vi "UI.vi"() -> ()   [LabVIEW 2018]
uses:
  lib/Tango/SubVIs/AxisControl.ctl
  <vilib>/MakerHub/LINX/Public/Utilities/Open Serial.vi
  lib/Olympus IX BX Series/Olympus IX BX Series.lvlib
  <vilib>/MakerHub/LINX/LMH-LINX.lvlib
  lib/SOLA/LabVIEW 2015 Library (32bit)/LumencorDLL32/LumencorDLL32.lvlib
panel:
  in  "SOLA COM Port":u32=5 max=10 step=1
  in  "Light Source":u16(ring) items=["BF - Lamp", "SOLA"]
  out "error out":errorcluster
  in  "Flush\nReagent":u16
  in  "Flush":bool
  in  "Pump Cycles":dbl=20.0
  in  "Frequency":dbl=50.0 format="%#_3f"
  in  "Pump On":bool
  in  "Feed On":bool
  in  "Feed Cycles":dbl=20.0
  in  "Feed\nReagent":u16=2
  in  "Ring":u16
  in  "All Rings":bool
  in  "Direction (1: Down)":enum16{"Up", "Down", "Abs"}(ring)=enum."Abs"
  in  "Step (0.0 um)":dbl format="%.1f"
  in  "Filter":enum32{"", "BF", "UV", "GFP", "YFP", "RFP"}(ring)=enum."RFP"
  in  "Prism Position (1: Bi)":enum16{"Bi", "Side"}(ring)=enum."Side"
  in  "Shutter":bool
  in  "Objective":T1(ring)=enum."x 4"
  in  "Intensity [%]":dbl(slide) scale=0.0..100.0 scale format="%.1f"
  in  "Enable Lamp":bool
  in  "Lamp Type (0: Transmitted)":enum16{"Transmitted", "Reflected"}(ring)
  in  "stop":bool
  in  "Valve Port (Arduino)":refnum<visa-resource-name>="COM7"
  in  "IX 81 Port (IX2 UCB)":refnum<visa-resource-name>="IX2-UCB"
  out "Upper Limit":dbl
  out "Lower Limit":dbl
  in  "Move absolute":bool
  in  "Destination [mm]":dbl[](array[numeric]) format="%_6g"
  in  "Manual Control":T2[](array[typedef])
  in  "Step Width [mm]":dbl=1.0 min=0.0 format="%_6f"
  out "Position":dbl[](array[numeric]) format="%_6f"
  in  "TANGO COM Port":refnum<visa-resource-name>="COM4"
  # "Valve Functions"
  # "Initialization"
  # "Microscope"
  # "Stage"
  # "X"
  # "Y"
  # "Z"
  # "A"
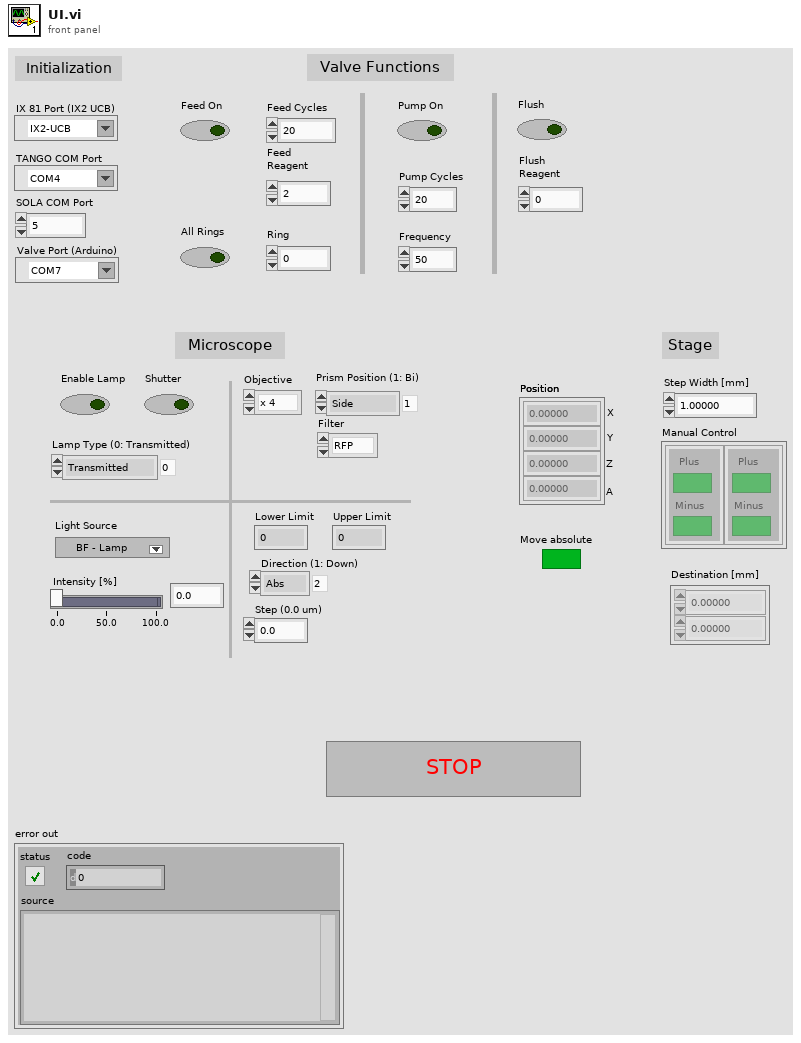
[diagram p1: front panel]
types:
  T1 = enum16{"", "x 4", "x 10", "x 20", "x 40", "x 100"}
  T2 = typedef "AxisControl.ctl" = cluster{"Plus":bool, "Minus":bool}
  T3 = typedef "LMH-LINX.lvlib/LINX Ref.ctl" = cluster{"IO":T4, "Interface":T5, "LINX Device Config":T6}
  T4 = typedef "LMH-LINX.lvlib/Platform.ctl" = enum16{"Remote", "Local"}
  T5 = typedef "LMH-LINX.lvlib/Interface.ctl" = enum16{"Serial", "TCP"}
  T6 = typedef "LMH-LINX.lvlib/Device.lvlib/LINX Device Config.ctl" = cluster{"Interface":T5, "COM Port":refnum<visa-resource-name>, "TCP Configuration":T7, "Device Family":u8, "Device ID":u8, "Device Name":string, "TCP Ref":refnum<k5>, "Channels":T8}
  T7 = typedef "LMH-LINX.lvlib/Device.lvlib/TCP Config.ctl" = cluster{"IP Address":string, "Port":u16}
  T8 = typedef "LMH-LINX.lvlib/Channels.ctl" = cluster{"DI":u8[], "DO":u8[], "AI":u8[], "AO":u8[], "PWM":u8[], "QE":u8[], "UART":u8[], "I2C 2":u8[], "SPI":u8[], "CAN":u8[], "Servo":u8[], "AI Ref (V)":dbl, "AI Resolution (Bits)":u8, "AO Ref (V)":dbl, "AO Resolution (Bits)":u8}
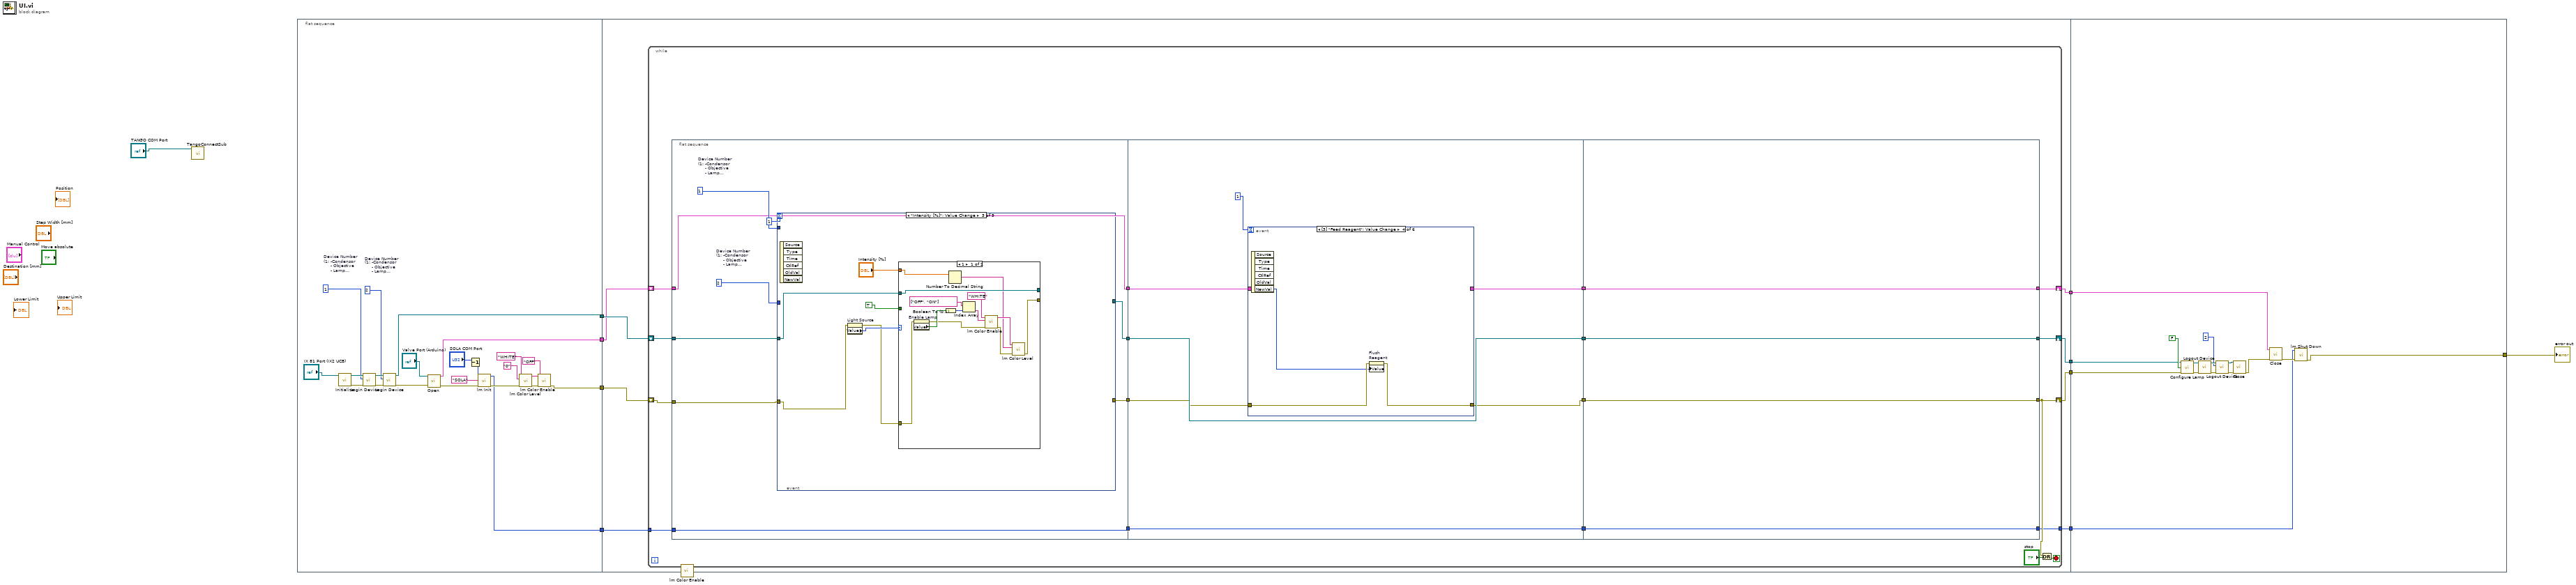
[diagram p0: block diagram]
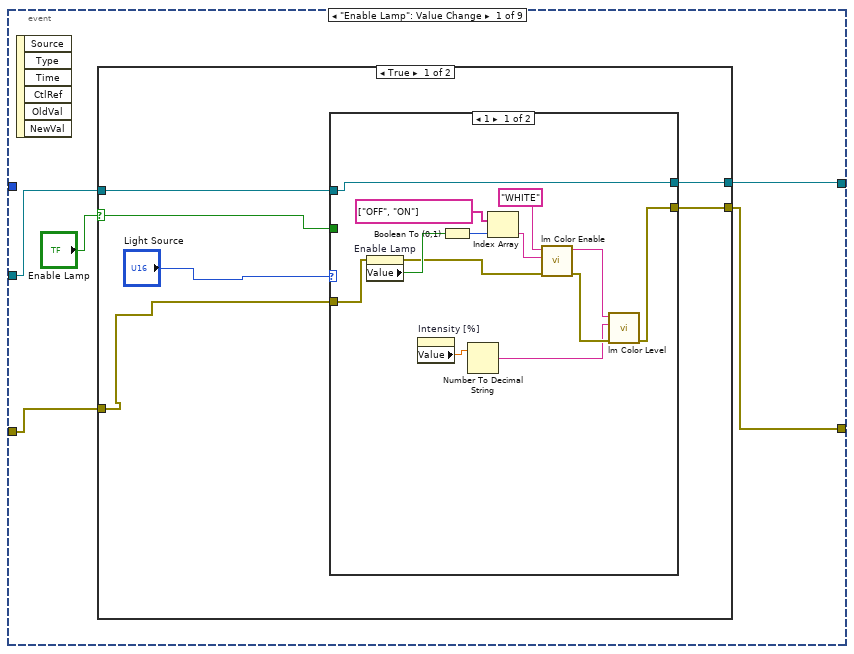
[diagram p2: hidden frame]
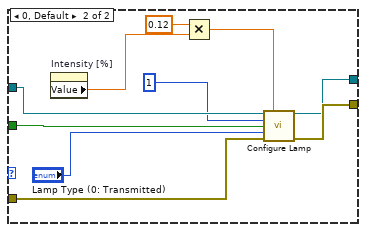
[diagram p3: hidden frame]
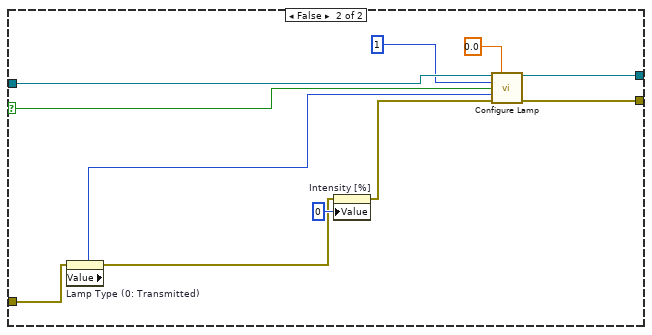
[diagram p4: hidden frame]
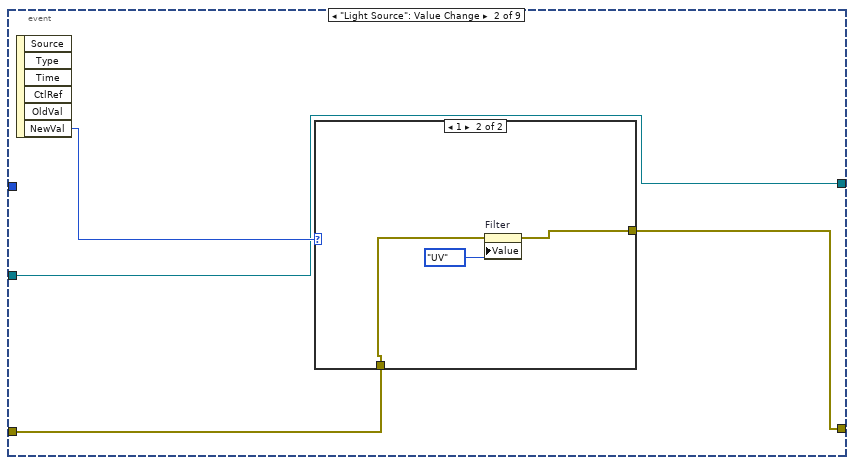
[diagram p5: hidden frame]
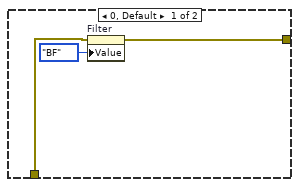
[diagram p6: hidden frame]
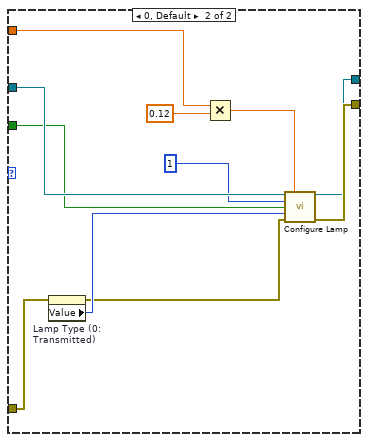
[diagram p7: hidden frame]
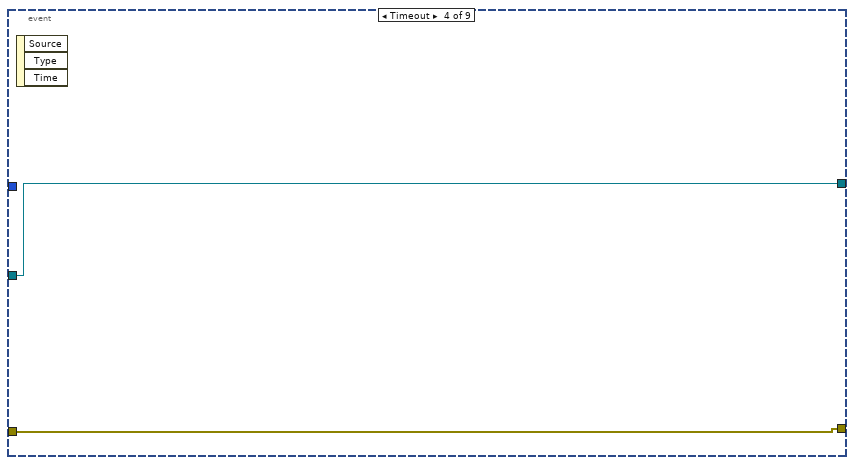
[diagram p8: hidden frame]
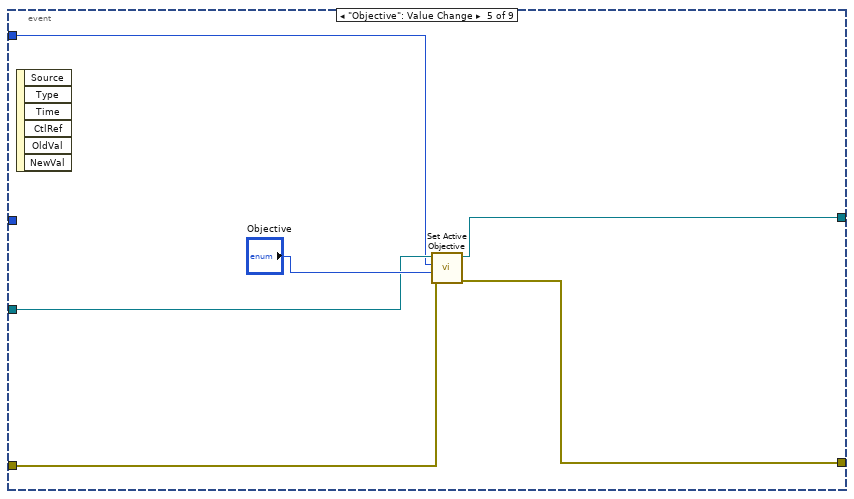
[diagram p9: hidden frame]
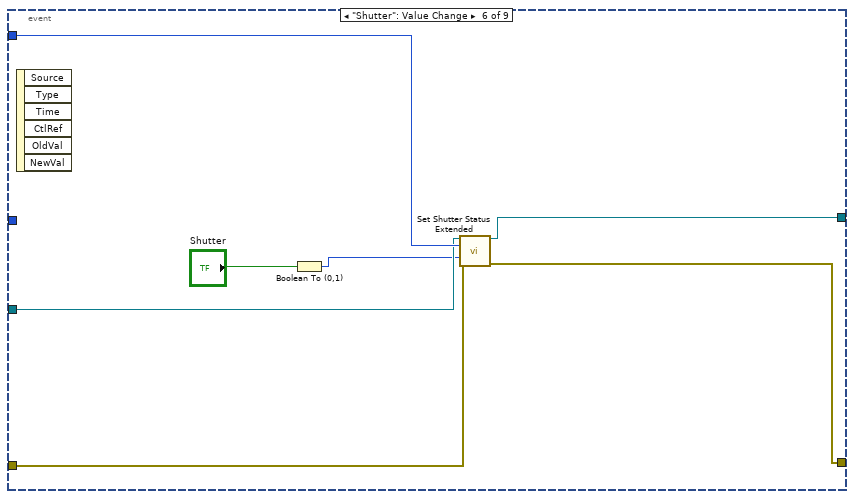
[diagram p10: hidden frame]
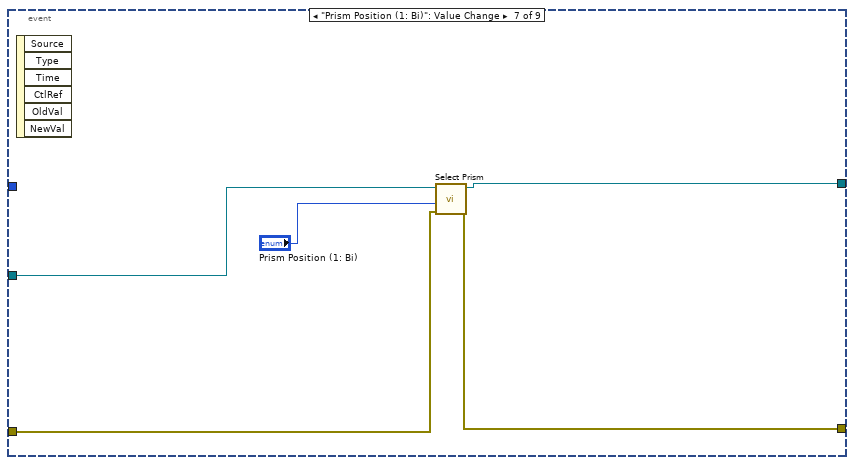
[diagram p11: hidden frame]
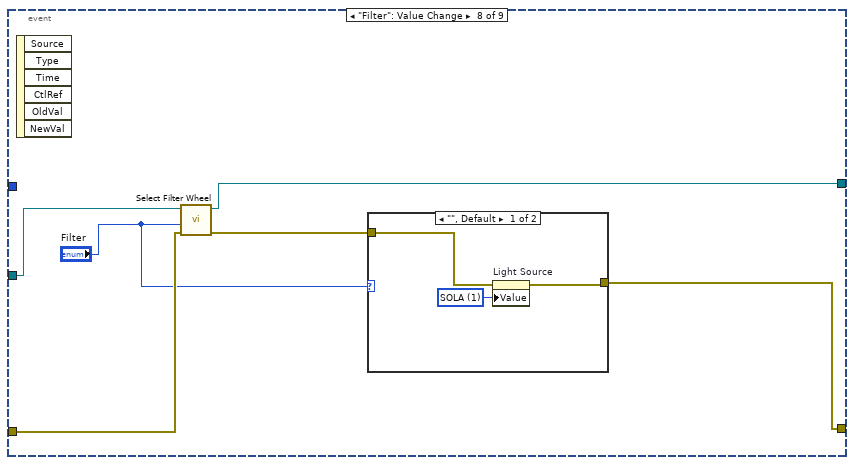
[diagram p12: hidden frame]
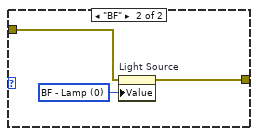
[diagram p13: hidden frame]
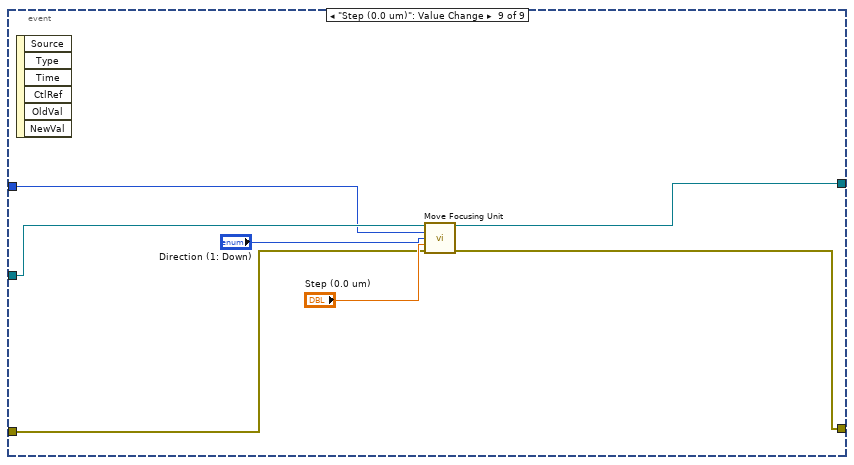
[diagram p14: hidden frame]
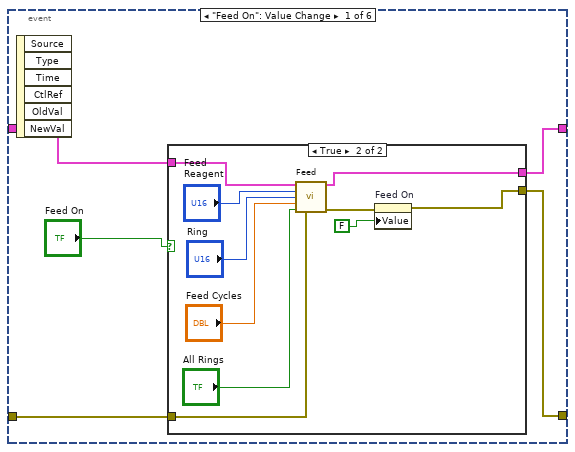
[diagram p15: hidden frame]
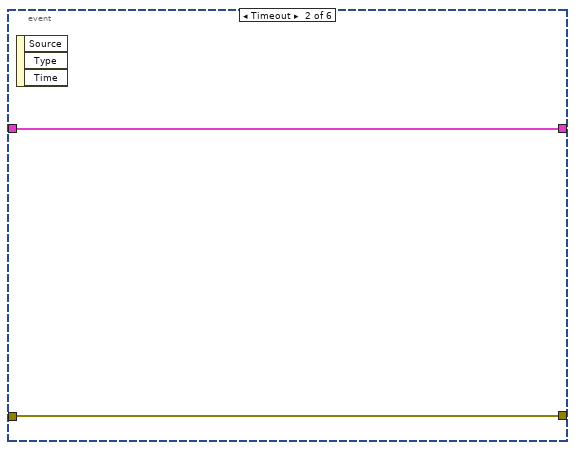
[diagram p17: hidden frame]
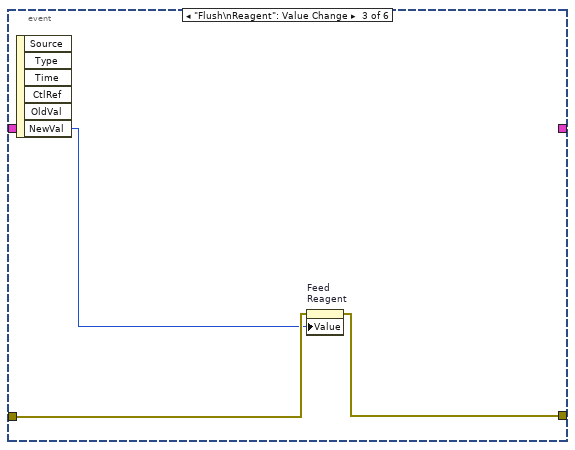
[diagram p18: hidden frame]
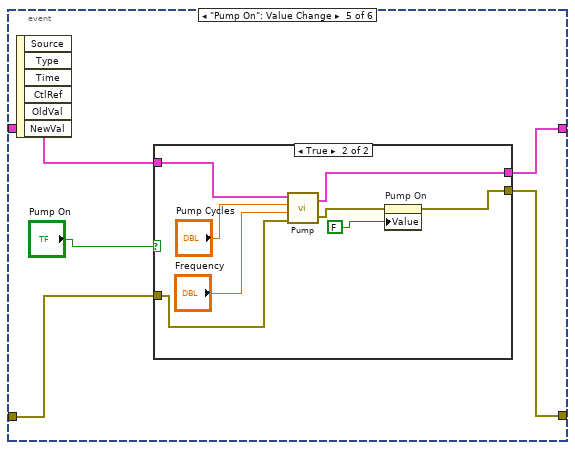
[diagram p19: hidden frame]
diagram:
  n1 = call "TangoConnectSub.vi"("VISA Refnum in"="TANGO COM Port") -> ()  [unwired: 8 in, 3 out]
  n2 = flat-sequence {
    tunnel: [w24] -> w9
    tunnel: [w23] -> w8
    tunnel: [w13] -> w7
    tunnel: [w12] -> w2
    tunnel: w9 -> [w41]
    tunnel: w8 -> [w39]
    tunnel: w7 -> [w40]
    tunnel: [w38] -> w6
    tunnel: [w37] -> w5
    tunnel: [w36] -> w4
    tunnel: w2 -> [w35]
    tunnel: [w34] -> w1
    tunnel: w6 -> [w261]
    tunnel: w5 -> [w260]
    tunnel: w4 -> [w259]
    tunnel: [w256] -> w3
    tunnel: w1 -> [w257]
    frame #0 {
      w26 = 2  # Device Number (1: -Condensor      - Objective      - Lamp      - Shutter 2: - Z-Motion    - Autofocus)
      w25 = 1  # Device Number (1: -Condensor      - Objective      - Lamp      - Shutter 2: - Z-Motion    - Autofocus)
      n3 = call "Initialize.vi"("VISA Resource Name"="IX 81 Port (IX2 UCB)") -> ("VISA Resource Name Out"=w32:refnum<visa-resource-name>, "error out"=w31:errorcluster)  [unwired: 13 in]
      n4 = call "Login Device.vi"("error in (no error)"=w31, "Device Number (1)"=w25, "VISA Resource Name"=w32) -> ("error out"=w29:errorcluster, "VISA Resource Name Out"=w30:refnum<visa-resource-name>)  [unwired: 7 in]
      n5 = call "Login Device.vi"("error in (no error)"=w29, "Device Number (1)"=w26, "VISA Resource Name"=w30) -> ("error out"=w27:errorcluster, "VISA Resource Name Out"=w24:refnum<visa-resource-name>)  [unwired: 7 in]
      n6 = call-poly <vilib>:"Open.vi"("Error In"=w27, "Serial Port"="Valve Port (Arduino)") -> ("Error Out"=w22:errorcluster, "LINX Resource"=w23:T3)  [unwired: 7 in, 1 out]
      n7 = Decrement(x="SOLA COM Port") -> (x-1=w11:u32)
      n8 = call "lm Init.vi"("error in (no error)"=w22, "LETypeStr"="SOLA", "ComPort"=w11) -> ("error out"=w19:errorcluster, "function return"=w12:u32)  [unwired: 6 in, 1 out]
      n9 = call "lm Color Level.vi"("error in (no error)"=w19, "str_Level"="0", "str_Color"="WHITE") -> ("error out"=w15:errorcluster, "str_Color out"=w16:string)  [unwired: 6 in, 1 out]
      n10 = call "lm Color Enable.vi"("error in (no error)"=w15, "str_State"="OFF", "str_Color"=w16) -> ("error out"=w13:errorcluster)  [unwired: 6 in, 2 out]
    }
    frame #1 {
      n11 = while {
        shift-right: [w46] -> w36
        shift-left: w40 -> [w56]
        shift-right: [w53] -> w38
        shift-left: w39 -> [w54]
        shift-right: [w55] -> w37
        shift-left: w41 -> [w57]
        tunnel: w35 -> [w45]
        tunnel: [w42] -> w34
        stop <- w58 stop-if-true
        n12 = flat-sequence {
          tunnel: w57 -> [w65]
          tunnel: w56 -> [w64]
          tunnel: [w63] -> w52
          tunnel: [w62] -> w51
          tunnel: w54 -> [w61]
          tunnel: [w61] -> w50
          tunnel: w45 -> [w60]
          tunnel: [w60] -> w44
          tunnel: w52 -> [w196]
          tunnel: [w196] -> w49
          tunnel: w51 -> [w195]
          tunnel: [w194] -> w48
          tunnel: w50 -> [w198]
          tunnel: [w197] -> w47
          tunnel: w44 -> [w193]
          tunnel: [w193] -> w43
          tunnel: [w254] -> w55
          tunnel: w49 -> [w254]
          tunnel: [w255] -> w46
          tunnel: w48 -> [w255]
          tunnel: [w253] -> w53
          tunnel: w47 -> [w253]
          tunnel: w43 -> [w252]
          tunnel: [w252] -> w42
          frame #0 {
            w66 = 2  # Device Number (1: -Condensor      - Objective      - Lamp      - Shutter 2: - Z-Motion    - Autofocus)
            w67 = 1  # Device Number (1: -Condensor      - Objective      - Lamp      - Shutter 2: - Z-Motion    - Autofocus)
            n13 = event shown="[2] \"Intensity [%]\": Value Change" {
              selector: _ -> [_ _ _ _ _ _ _ _ _]
              dyn-events: _ -> [_ _ _ _ _ _ _ _ _]
              timeout: 1 -> [_ _ _ _ _ _ _ _ _]
              tunnel: w65 -> [w72 w114 w128 w155 w158 w167 w170 w177 w189]
              tunnel: w67 -> [_ _ _ _ w156 w168 _ _ _]
              tunnel: w66 -> [_ _ _ _ _ _ _ _ w188]
              tunnel: [w71 w115 _ w154 w160 w162 w172 w174 w186] -> w62
              tunnel: [w70 w114 _ w155 w161 w163 w173 w179 w187] -> w63
              tunnel: w64 -> [w69 w116 w126 w154 w157 w166 w171 w178 w190]
              event "Enable Lamp": Value Change {
                n14 = event-data() -> ()  [unwired: 1 in, 6 out]
                n15 = case shown="True" "Enable Lamp" {
                  selector: "Enable Lamp" -> [w76 w109]
                  tunnel: w72 -> [w79 w113]
                  tunnel: w69 -> [w75 w104]
                  tunnel: [w78 w112] -> w71
                  tunnel: [w77 w111] -> w70
                  frame True {
                    n16 = case shown="1" "Light Source" {
                      tunnel: w79 -> [w92 w102]
                      tunnel: w75 -> [w86 w101]
                      tunnel: [w80 w100] -> w78
                      tunnel: [w92 w99] -> w77
                      tunnel: w76 -> [_ w97]
                      frame 1 {
                        n17 = property on="Enable Lamp" class="Bool (strict)"(error in=w86) -> (error out=w85:errorcluster, "Value"=w88:bool)  [unwired: 1 in, 1 out]
                        n18 = property on="Intensity [%]" class="Slide (strict)"() -> ("Value"=w82:dbl)  [unwired: 2 in, 2 out]
                        n19 = Boolean To (0,1)(Boolean=w88) -> (0, 1=w87:i16)
                        n20 = Number To Decimal String(number=w82) -> (decimal integer string=w81:string)  [unwired: 1 in]
                        n21 = Index Array(array=string[] ["OFF", "ON"], index=w87) -> (element=w90:string)
                        n22 = call "lm Color Enable.vi"("error in (no error)"=w85, "str_State"=w90, "str_Color"="WHITE") -> ("error out"=w84:errorcluster, "str_Color out"=w83:string)  [unwired: 6 in, 1 out]
                        n23 = call "lm Color Level.vi"("error in (no error)"=w84, "str_Level"=w81, "str_Color"=w83) -> ("error out"=w80:errorcluster)  [unwired: 6 in, 2 out]
                      }
                      frame 0, Default {
                        n24 = property on="Intensity [%]" class="Slide (strict)"() -> ("Value"=w94:dbl)  [unwired: 2 in, 2 out]
                        n25 = Multiply(x=0.12, y=w94) -> (x*y=w96:dbl)
                        n26 = call "Configure Lamp.vi"("VISA Resource Name"=w102, "Lamp Intensity (1.0 V)"=w96, "Device Number (1)"=1, "Lamp Enabled (True)"=w97, "Lamp Type (0: Transmitted)"="Lamp Type (0: Transmitted)", "error in (no error)"=w101) -> ("VISA Resource Name Out"=w99:refnum<visa-resource-name>, "error out"=w100:errorcluster)  [unwired: 8 in]
                      }
                    }
                  }
                  frame False {
                    n27 = property on="Lamp Type (0: Transmitted)" class="Enum (strict)"(error in=w104) -> (error out=w103:errorcluster, "Value"=w105:enum16{"Transmitted", "Reflected"})  [unwired: 1 in, 1 out]
                    n28 = property on="Intensity [%]" class="Slide (strict)"(error in=w103, "Value"=u16 0 ("Intensity [%]")) -> (error out=w108:errorcluster)  [unwired: 1 in, 1 out]
                    n29 = call "Configure Lamp.vi"("VISA Resource Name"=w113, "Lamp Intensity (1.0 V)"=0.0, "Device Number (1)"=1, "Lamp Enabled (True)"=w109, "Lamp Type (0: Transmitted)"=w105, "error in (no error)"=w108) -> ("VISA Resource Name Out"=w111:refnum<visa-resource-name>, "error out"=w112:errorcluster)  [unwired: 8 in]
                  }
                }
              }
              event "Light Source": Value Change {
                n30 = event-data() -> ("NewVal"=w117:u16)  [unwired: 1 in, 5 out]
                n31 = case shown="1" w117 {
                  tunnel: w116 -> [w119 w122]
                  tunnel: [w118 w121] -> w115
                  frame 0, Default {
                    n32 = property on="Filter" class="Enum (strict)"(error in=w119, "Value"=enum32{"", "BF", "UV", "GFP", "YFP", "RFP"}."BF" ("Filter")) -> (error out=w118:errorcluster)  [unwired: 1 in, 1 out]
                  }
                  frame 1 {
                    n33 = property on="Filter" class="Enum (strict)"(error in=w122, "Value"=enum32{"", "BF", "UV", "GFP", "YFP", "RFP"}."UV" ("Filter")) -> (error out=w121:errorcluster)  [unwired: 1 in, 1 out]
                  }
                }
              }
              event "Intensity [%]": Value Change {
                n34 = event-data() -> ()  [unwired: 1 in, 6 out]
                n35 = property on="Light Source" class="Ring (strict)"(error in=w126) -> (error out=w125:errorcluster, "Value"=w129:u16)  [unwired: 1 in, 1 out]
                n36 = case shown="1" w129 {
                  tunnel: w128 -> [w142 w153]
                  tunnel: [w132 w152] -> _
                  tunnel: [w142 w151] -> _
                  tunnel: TRUE -> [_ w149]
                  tunnel: w125 -> [w131 w146]
                  tunnel: "Intensity [%]" -> [w130 w144]
                  frame 1 {
                    n37 = property on="Enable Lamp" class="Bool (strict)"(error in=w131) -> (error out=w136:errorcluster, "Value"=w138:bool)  [unwired: 1 in, 1 out]
                    n38 = Boolean To (0,1)(Boolean=w138) -> (0, 1=w137:i16)
                    n39 = Number To Decimal String(number=w130) -> (decimal integer string=w133:string)  [unwired: 1 in]
                    n40 = Index Array(array=string[] ["OFF", "ON"], index=w137) -> (element=w140:string)
                    n41 = call "lm Color Enable.vi"("error in (no error)"=w136, "str_State"=w140, "str_Color"="WHITE") -> ("error out"=w135:errorcluster, "str_Color out"=w134:string)  [unwired: 6 in, 1 out]
                    n42 = call "lm Color Level.vi"("error in (no error)"=w135, "str_Level"=w133, "str_Color"=w134) -> ("error out"=w132:errorcluster)  [unwired: 6 in, 2 out]
                  }
                  frame 0, Default {
                    n43 = property on="Lamp Type (0: Transmitted)" class="Enum (strict)"(error in=w146) -> (error out=w145:errorcluster, "Value"=w147:enum16{"Transmitted", "Reflected"})  [unwired: 1 in, 1 out]
                    n44 = Multiply(x=w144, y=0.12 ("x")) -> (x*y=w148:dbl)
                    n45 = call "Configure Lamp.vi"("VISA Resource Name"=w153, "Lamp Intensity (1.0 V)"=w148, "Device Number (1)"=1, "Lamp Enabled (True)"=w149, "Lamp Type (0: Transmitted)"=w147, "error in (no error)"=w145) -> ("VISA Resource Name Out"=w151:refnum<visa-resource-name>, "error out"=w152:errorcluster)  [unwired: 8 in]
                  }
                }
              }
              event Timeout {
                n46 = event-data() -> ()  [unwired: 1 in, 3 out]
              }
              event "Objective": Value Change {
                n47 = event-data() -> ()  [unwired: 1 in, 6 out]
                n48 = call "Set Active Objective.vi"("error in (no error)"=w157, "Objective Number (1)"="Objective", "Device Number (1)"=w156, "VISA Resource Name"=w158) -> ("error out"=w160:errorcluster, "VISA Resource Name Out"=w161:refnum<visa-resource-name>)  [unwired: 6 in]
              }
              event "Shutter": Value Change {
                n49 = event-data() -> ()  [unwired: 1 in, 6 out]
                n50 = Boolean To (0,1)(Boolean="Shutter") -> (0, 1=w164:i16)
                n51 = call "Set Shutter Status Extended.vi"("VISA Resource Name"=w167, "Device Number (1)"=w168, "Shutter Status (0: Open)"=w164, "error in (no error)"=w166) -> ("VISA Resource Name Out"=w163:refnum<visa-resource-name>, "error out"=w162:errorcluster)  [unwired: 10 in]
              }
              event "Prism Position (1: Bi)": Value Change {
                n52 = event-data() -> ()  [unwired: 1 in, 6 out]
                n53 = call "Select Prism.vi"("error in (no error)"=w171, "Prism Position (0: Bi)"="Prism Position (1: Bi)", "VISA Resource Name"=w170) -> ("error out"=w172:errorcluster, "VISA Resource Name Out"=w173:refnum<visa-resource-name>)  [unwired: 7 in]
              }
              event "Filter": Value Change {
                n54 = event-data() -> ()  [unwired: 1 in, 6 out]
                n55 = call "Select Filter Wheel.vi"("error in (no error)"=w178, "Filter Wheel Position (1)"="Filter", "VISA Resource Name"=w177) -> ("error out"=w175:errorcluster, "VISA Resource Name Out"=w179:refnum<visa-resource-name>)  [unwired: 7 in]
                n56 = case shown="\"\", Default" "Filter" {
                  tunnel: w175 -> [w180 w185]
                  tunnel: [w181 w184] -> w174
                  frame "", Default {
                    w182 = u16 1 items=["BF - Lamp", "SOLA"] ("Light Source")
                    n57 = property on="Light Source" class="Ring (strict)"(error in=w180, "Value"=w182) -> (error out=w181:errorcluster)  [unwired: 1 in, 1 out]
                  }
                  frame "BF" {
                    w183 = u16 0 items=["BF - Lamp", "SOLA"] ("Light Source")
                    n58 = property on="Light Source" class="Ring (strict)"(error in=w185, "Value"=w183) -> (error out=w184:errorcluster)  [unwired: 1 in, 1 out]
                  }
                }
              }
              event "Step (0.0 um)": Value Change {
                n59 = event-data() -> ()  [unwired: 1 in, 6 out]
                n60 = call "Move Focusing Unit.vi"("VISA Resource Name"=w189, "Device Number (1)"=w188, "Direction (1: Down)"="Direction (1: Down)", "Step (0.0 um)"="Step (0.0 um)", "error in (no error)"=w190) -> ("VISA Resource Name Out"=w187:refnum<visa-resource-name>, "error out"=w186:errorcluster)  [unwired: 9 in]
              }
            }
          }
          frame #1 {
            n61 = event shown="[3] \"Feed Reagent\": Value Change" {
              selector: _ -> [_ _ _ _ _ _]
              dyn-events: _ -> [_ _ _ _ _ _]
              timeout: 1 -> [_ _ _ _ _ _]
              tunnel: w195 -> [w204 w217 w221 w224 w229 w244]
              tunnel: w198 -> [w203 w218 _ _ w228 w243]
              tunnel: [w201 w217 w220 w223 w226 w241] -> w194
              tunnel: [w200 w218 _ _ w227 w242] -> w197
              event "Feed On": Value Change {
                n62 = event-data() -> ()  [unwired: 1 in, 6 out]
                n63 = case shown="True" "Feed On" {
                  tunnel: w204 -> [w205 w216]
                  tunnel: w203 -> [w206 w215]
                  tunnel: [w205 w213] -> w201
                  tunnel: [w206 w207] -> w200
                  frame False {
                  }
                  frame True {
                    n64 = call "Feed.vi"("LINX Resource"=w215, "Channel"="Feed\nReagent", "Ring"="Ring", "Feed Cycles"="Feed Cycles", "All Rings"="All Rings", "error in (no error)"=w216) -> ("LINX Resource out"=w207:T3, "error out"=w214:errorcluster)  [unwired: 8 in]
                    n65 = property on="Feed On" class="Bool (strict)"(error in=w214, "Value"=FALSE) -> (error out=w213:errorcluster)  [unwired: 1 in, 1 out]
                  }
                }
              }
              event Timeout {
                n66 = event-data() -> ()  [unwired: 1 in, 3 out]
              }
              event "Flush\nReagent": Value Change {
                n67 = event-data() -> ("NewVal"=w219:u16)  [unwired: 1 in, 5 out]
                n68 = property on="Feed\nReagent" class="DigNum (strict)"(error in=w221, "Value"=w219) -> (error out=w220:errorcluster)  [unwired: 1 in, 1 out]
              }
              event "Feed\nReagent": Value Change {
                n69 = event-data() -> ("NewVal"=w222:u16)  [unwired: 1 in, 5 out]
                n70 = property on="Flush\nReagent" class="DigNum (strict)"(error in=w224, "Value"=w222) -> (error out=w223:errorcluster)  [unwired: 1 in, 1 out]
              }
              event "Pump On": Value Change {
                n71 = event-data() -> ()  [unwired: 1 in, 6 out]
                n72 = case shown="True" "Pump On" {
                  tunnel: w229 -> [w230 w234]
                  tunnel: w228 -> [w231 w237]
                  tunnel: [w230 w239] -> w226
                  tunnel: [w231 w232] -> w227
                  frame False {
                  }
                  frame True {
                    n73 = call "Pump.vi"("error in (no error)"=w234, "Pump Frequency"="Frequency", "Pump Cycles"="Pump Cycles", "LINX Resource"=w237) -> ("error out"=w233:errorcluster, "LINX Resource out"=w232:T3)
                    n74 = property on="Pump On" class="Bool (strict)"(error in=w233, "Value"=FALSE) -> (error out=w239:errorcluster)  [unwired: 1 in, 1 out]
                  }
                }
              }
              event "Flush": Value Change {
                n75 = event-data() -> ()  [unwired: 1 in, 6 out]
                n76 = case shown="True" "Flush" {
                  tunnel: w244 -> [w245 w249]
                  tunnel: w243 -> [w246 w251]
                  tunnel: [w245 w248] -> w241
                  tunnel: [w246 w247] -> w242
                  frame False {
                  }
                  frame True {
                    n77 = call "Flush.vi"("error in (no error)"=w249, "Channel"="Flush\nReagent", "LINX Resource"=w251) -> ("error out"=w248:errorcluster, "LINX Resource out"=w247:T3)  [unwired: 7 in]
                  }
                }
              }
            }
          }
          frame #2 {
          }
        }
        n78 = Or(x=w46, y="stop") -> (x .or. y?=w58:bool)
      }
    }
    frame #2 {
      n79 = call "Configure Lamp.vi"("VISA Resource Name"=w260, "Lamp Enabled (True)"=FALSE, "error in (no error)"=w259) -> ("VISA Resource Name Out"=w265:refnum<visa-resource-name>, "error out"=w266:errorcluster)  [unwired: 11 in]
      n80 = call "Logout Device.vi"("error in (no error)"=w266, "VISA Resource Name"=w265) -> ("error out"=w268:errorcluster, "VISA Resource Name Out"=w267:refnum<visa-resource-name>)  [unwired: 8 in]
      n81 = call "Logout Device.vi"("error in (no error)"=w268, "Device Number (1)"=2, "VISA Resource Name"=w267) -> ("error out"=w270:errorcluster, "VISA Resource Name Out"=w269:refnum<visa-resource-name>)  [unwired: 7 in]
      n82 = call <vilib>:"Close.vi"("VISA Resource Name"=w269, "error in (no error)"=w270) -> ("error out"=w262:errorcluster)  [unwired: 13 in]
      n83 = call <vilib>:"Close.vi"("Error In"=w262, "LINX Resource"=w261) -> ("Error Out"=w258:errorcluster)  [unwired: 9 in]
      n84 = call "lm Shut Down.vi"("error in (no error)"=w258, "hSerial"=w257) -> ("error out"=w256:errorcluster)  [unwired: 8 in, 1 out]
    }
  }
  n85 = call "lm Color Enable.vi"() -> ()  [unwired: 9 in, 3 out]
  "error out" <- w3
